vi "Connection Loop.vi"(8 "error in (no error)":errorcluster, 11 "TCP Comm":T2) -> (0 "error out":errorcluster)   [LabVIEW 2020, in "TinyTCP.lvlib"]
uses:
  TinyTCP.lvlib
  Instance.ctl
  Ref Data.ctl
  State.ctl
panel:
  out "local-port":u16 caption="local/incoming-port"
  out "Certificate DN":string
  out "TLS Enabled":bool
  out "Server":bool
  out "Port":u16
  out "Host":string
  out "State":T1
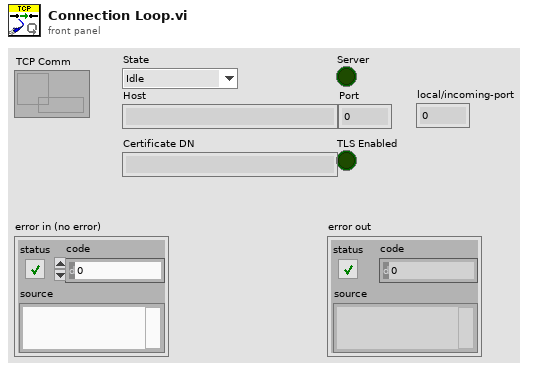
[diagram p1: front panel]
types:
  T1 = typedef "TinyTCP.lvlib/State.ctl" = enum16{"Idle", "Starting", "Connecting", "Connected", "Disconnecting", "Stopped"}
  T2 = typedef "TinyTCP.lvlib/Instance.ctl" = refnum<data-value>
  T3 = typedef "TinyTCP.lvlib/Ref Data.ctl" = cluster{"TCP":refnum<k5>, "State":T1, "Server":bool, "Host":string, "Port":u16, "Listener":refnum<k5>, "Start":bool, "Disconnect":bool, "TCP Valid":bool, "TLS Enabled":bool, "Immutable TLS":refnum<k36>, "Certificate DN":string, "local-port":u16}
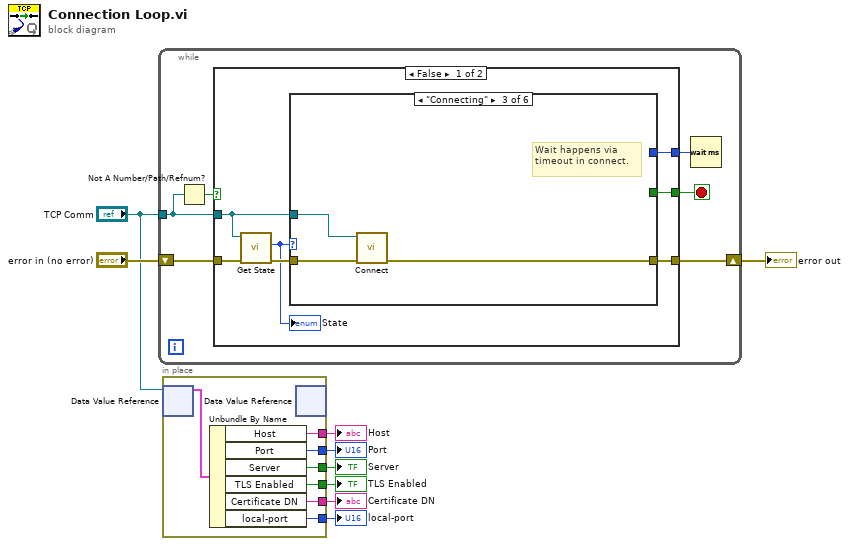
[diagram p0: block diagram]
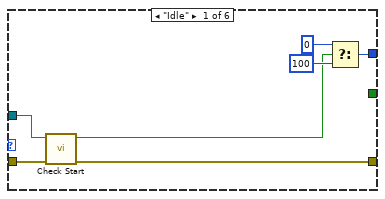
[diagram p2: hidden frame]
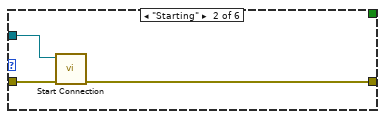
[diagram p3: hidden frame]
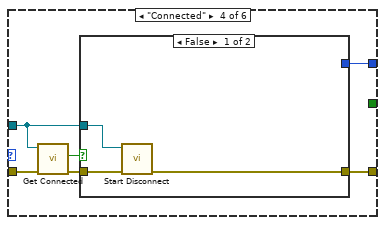
[diagram p4: hidden frame]
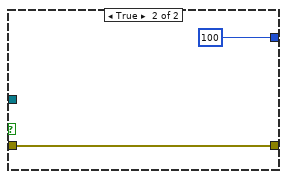
[diagram p5: hidden frame]
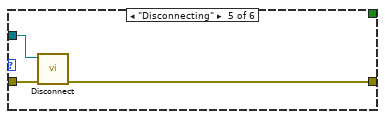
[diagram p6: hidden frame]
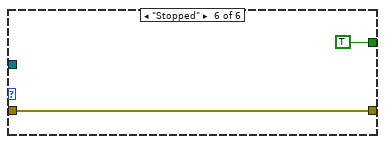
[diagram p7: hidden frame]
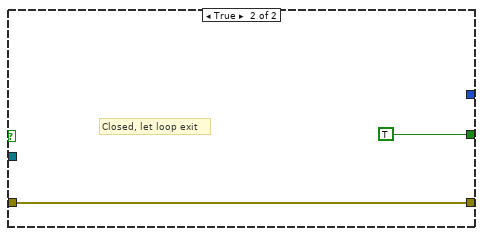
[diagram p8: hidden frame]
diagram:
  n1 = while {
    shift-right: [w10] -> w8
    shift-left: "error in (no error)" -> [w13]
    tunnel: "TCP Comm" -> [w14]
    stop <- w12 stop-if-true
    n2 = Not A Number/Path/Refnum?(number/path/refnum=w14) -> (NaN/Path/Refnum?=w15:bool)
    n3 = case shown="False" w15 {
      tunnel: w14 -> [w20 _]
      tunnel: w13 -> [w19 w52]
      tunnel: [w17 TRUE] -> w12
      tunnel: [w22 _] -> w11
      tunnel: [w21 w52] -> w10
      frame False {
        n4 = call "Get State.vi"("error in (no error)"=w19, "TCP Comm In"=w20) -> ("error out"=w18:errorcluster, "State"=w16:T1)  [unwired: 8 in]
        "State" <- w16
        n5 = case shown="\"Connecting\"" w16 {
          tunnel: [w23 _ _ w37 _ _] -> w22
          tunnel: w18 -> [w27 w31 w34 w41 w49 w51]
          tunnel: [w25 w30 w33 w36 w47 w51] -> w21
          tunnel: w20 -> [w26 w32 w35 w38 w48 _]
          tunnel: [_ _ _ _ _ TRUE] -> w17
          frame "Idle" {
            n6 = call "Check Start.vi"("error in (no error)"=w27, "TCP Comm"=w26) -> ("error out"=w25:errorcluster, "Start"=w24:bool)  [unwired: 8 in]
            n7 = Select(t=u32 0 ("milliseconds to wait"), s=w24, f=u32 100 ("milliseconds to wait")) -> (s? t:f=w23:u32)
          }
          frame "Starting" {
            n8 = call "Start Connection.vi"("error in (no error)"=w31, "TCP Comm"=w32) -> ("error out"=w30:errorcluster)  [unwired: 9 in]
          }
          frame "Connecting" {
            # "Wait happens via timeout in connect."
            n9 = call "Connect.vi"("error in (no error)"=w34, "TCP Comm"=w35) -> ("error out"=w33:errorcluster)  [unwired: 9 in]
          }
          frame "Connected" {
            n10 = call "Get Connected.vi"("error in (no error)"=w41, "TCP Comm"=w38) -> ("error out"=w40:errorcluster, "Connected"=w39:bool)  [unwired: 8 in]
            n11 = case shown="False" w39 {
              tunnel: w40 -> [w44 w45]
              tunnel: w38 -> [w43 _]
              tunnel: [_ u32 100 ("milliseconds to wait")] -> w37
              tunnel: [w42 w45] -> w36
              frame False {
                n12 = call "Start Disconnect.vi"("error in (no error)"=w44, "TCP Comm"=w43) -> ("error out"=w42:errorcluster)  [unwired: 9 in]
              }
              frame True {
              }
            }
          }
          frame "Disconnecting" {
            n13 = call "Disconnect.vi"("error in (no error)"=w49, "TCP Comm"=w48) -> ("error out"=w47:errorcluster)  [unwired: 9 in]
          }
          frame "Stopped" {
          }
        }
      }
      frame True {
        # "Closed, let loop exit"
      }
    }
    n14 = Wait (ms)(milliseconds to wait=w11) -> ()  [unwired: 1 out]
  }
  "error out" <- w8
  n15 = in-place {
    in-place-border: [w59] -> w6
    in-place-border: [w58] -> w5
    in-place-border: [w57] -> w4
    in-place-border: [w56] -> w3
    in-place-border: [w55] -> w2
    in-place-border: [w54] -> w1
    n16 = in-place-dvr #1("TCP Comm") -> (w60:T3)  [unwired: 1 out]
    n17 = Unbundle By Name(w60) -> ("Host"=w59:string, "Port"=w58:u16, "Server"=w57:bool, "TLS Enabled"=w56:bool, "Certificate DN"=w55:string, "local-port"=w54:u16)
    n18 = in-place-dvr #1() -> ()  [unwired: 1 in, 2 out]
  }
  "Host" <- w6
  "Port" <- w5
  "Server" <- w4
  "TLS Enabled" <- w3
  "Certificate DN" <- w2
  "local-port" <- w1
